vi "Split Lines.vi"(8 "error in (no error)":errorcluster, 10 "spreadsheet string":string, 11 "Construct String Setup Cam in":refnum<class "Construct String Setup Cam.lvclass">) -> (0 "error out":errorcluster, 2 "array":string[](array[string]), 3 "Construct String Setup Cam out":refnum<class "Construct String Setup Cam.lvclass">)   [LabVIEW 2018, in "Construct String Setup Cam.lvclass"]
doc: "Este VI recebe uma string e retorna um array onde cada elemento contém uma das linhas da string."
uses:
  Construct String Setup Cam.lvclass
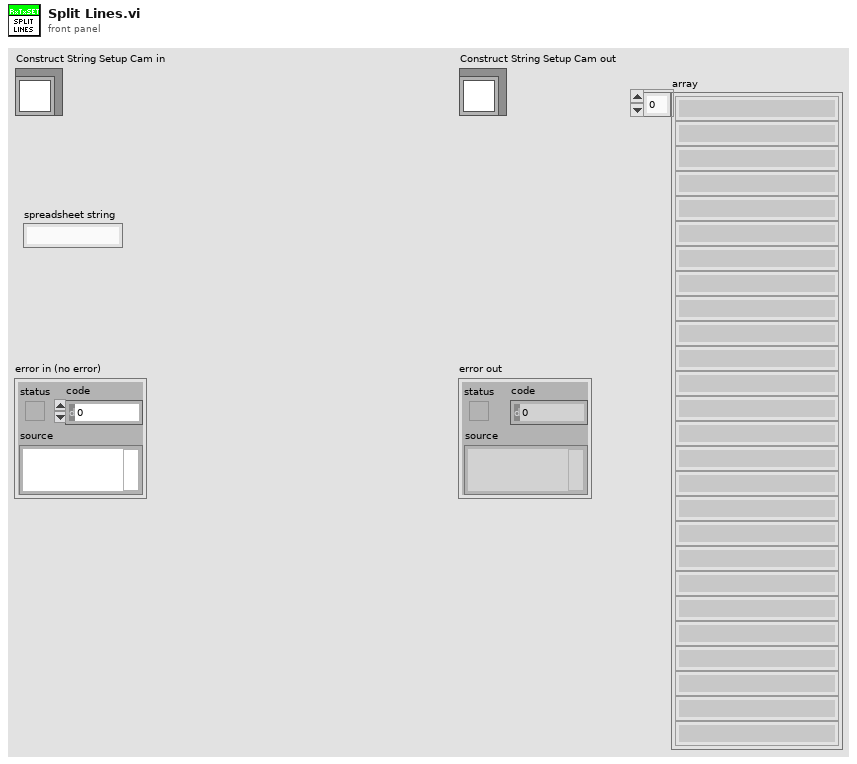
[diagram p1: front panel]
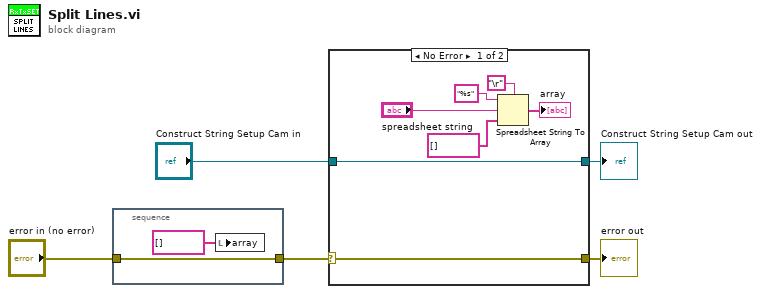
[diagram p0: block diagram]
diagram:
  n1 = stacked-sequence {
    tunnel: "error in (no error)" -> [w6]
    tunnel: [w6] -> w1
    frame #0 {
      n2 = local write "array"(string[] []) -> ()
    }
  }
  n3 = case shown="No Error" w1 {
    selector: w1 -> [w13 w16]
    tunnel: [w13 w16] -> w5
    tunnel: [w14 w15] -> w3
    tunnel: "Construct String Setup Cam in" -> [w14 w15]
    frame No Error {
      n4 = Spreadsheet String To Array(delimiter (Tab)="\r", format string="%s", spreadsheet string="spreadsheet string", array type (2D Dbl)=string[] []) -> (array=→"array":string[])
    }
    frame Error {
    }
  }
  "error out" <- w5
  "Construct String Setup Cam out" <- w3
